vi "Compute DistanceToTargetALG.vi"(10 "Line":T1, 11 "Image Src":T2) -> (1 "Angle to Target":dbl, 2 "Distance (ft)":dbl, 3 "Image Dst Out":T2)   [LabVIEW 2023]
doc: "Using the camera lens information and the real world size of the target, use trig and ratios to determine the distance to the target. Also returns the location relative to the image center in a (-1 , 1) coordinate system that may be useful for steering the robot."
uses:
  <vilib>/vision/Image Controls.llb/IMAQ Image.ctl
panel:
  out "Normalized Angle":dbl
  in  "X FOV":dbl=320.0 format="%#_13g"
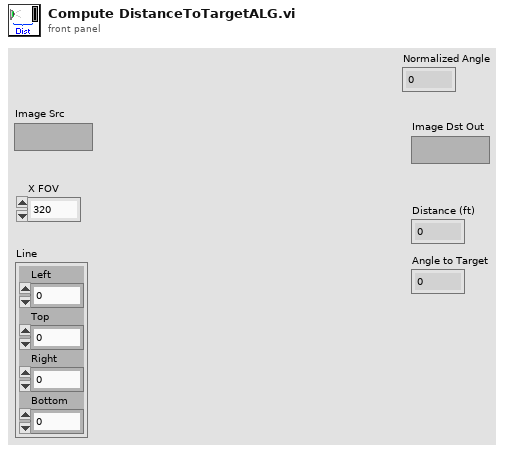
[diagram p1: front panel]
types:
  T1 = cluster{"Left":dbl, "Top":dbl, "Right":dbl, "Bottom":dbl}
  T2 = typedef "IMAQ Image.ctl" = refnum<image>
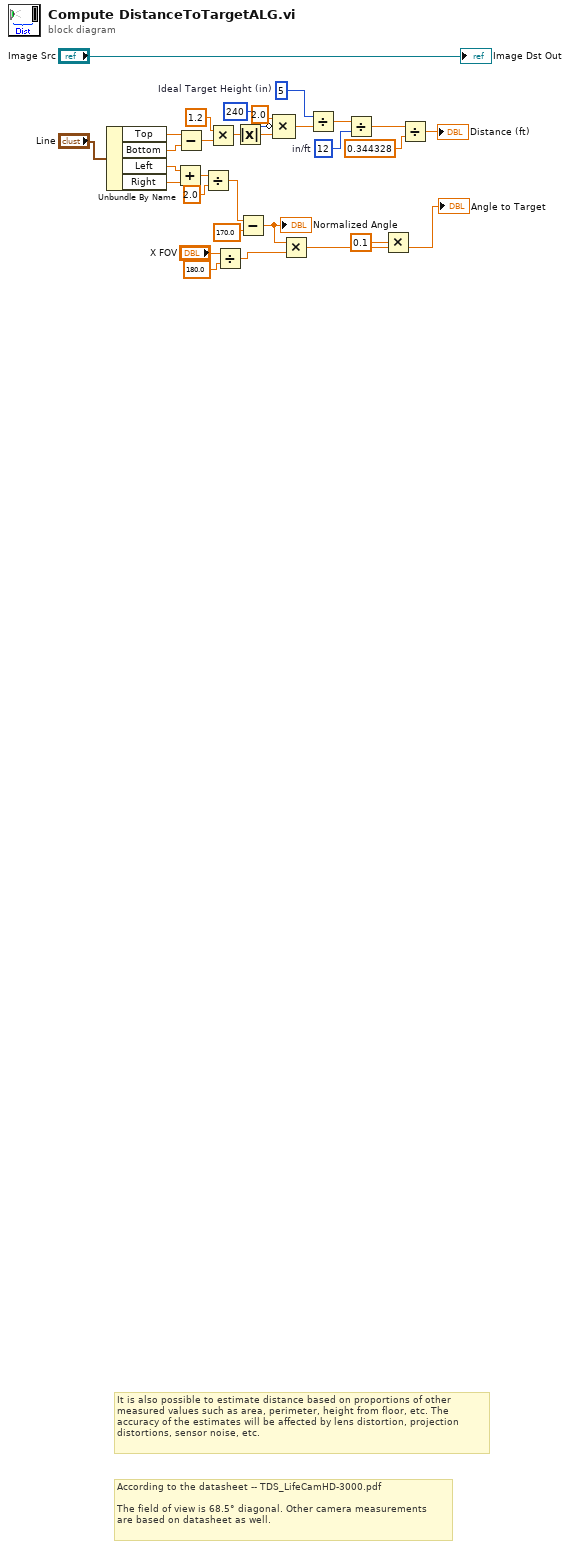
[diagram p0: block diagram]
diagram:
  w26 = 5  # Ideal Target Height (in)
  w30 = 12  # in/ft
  # "It is also possible to estimate distance based on proportions of other\nmeasured values such as area, perimeter, height from floor, etc. The\naccuracy of the estimates will be affected by lens distortion, projection\ndistortions, sensor noise, etc."
  # "According to the datasheet -- TDS_LifeCamHD-3000.pdf\n\nThe field of view is 68.5° diagonal. Other camera measurements\nare based on datasheet as well."
  n1 = Unbundle By Name("Line") -> ("Top"=w23:dbl, "Bottom"=w22:dbl, "Left"=w12:dbl, "Right"=w11:dbl)
  n2 = Add(x=w12, y=w11) -> (x+y=w10:dbl)
  n3 = Subtract(x=w23, y=w22) -> (x-y=w20:dbl)
  n4 = Divide(x=w10, y=2.0) -> (x/y=w6:dbl)
  n5 = Multiply(x=1.2, y=w20) -> (x*y=w19:dbl)
  n6 = Divide(x="X FOV", y=180.0) -> (x/y=w4:dbl)
  n7 = Absolute Value(x=w19) -> (abs(x)=w21:dbl)
  n8 = Subtract(x=w6, y=170.0) -> (x-y=w5:dbl)
  "Normalized Angle" <- w5
  n9 = Compound Arithmetic op=MULTIPLY(2.0, invert 240 ("Y Resolution"), w21) -> (w24:dbl)
  n10 = Multiply(x=w5, y=w4) -> (x*y=w3:dbl)
  n11 = Divide(x=w26, y=w24) -> (x/y=w28:dbl)
  n12 = Divide(x=w28, y=w30) -> (x/y=w27:dbl)
  n13 = Multiply(x=0.1, y=w3) -> (x*y=→"Angle to Target":dbl)
  n14 = Divide(x=w27, y=0.344328 ("FOV")) -> (x/y=→"Distance (ft)":dbl)
  "Image Dst Out" <- "Image Src"
